vi "Logging List Tree Items.vi"(3 "TreeRef":refnum<vi>) -> (0 "Items":string[](array[string]), 1 "TreeRef":refnum<vi>)   [LabVIEW 2012, in "femtoRoboLib.lvlib"]
uses:
  femtoRoboLib.lvlib
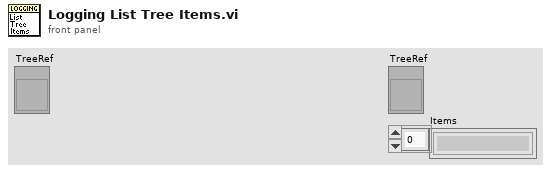
[diagram p1: front panel]
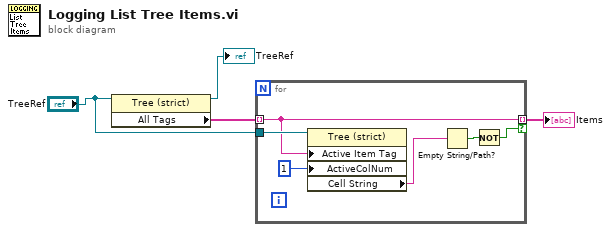
[diagram p0: block diagram]
diagram:
  n1 = property class="Tree (strict)"(reference="TreeRef") -> (reference out=→"TreeRef":refnum<vi>, "All Tags"=w3:string[])  [unwired: 1 in, 1 out]
  n2 = for {
    tunnel: w3 -> [w9] mode=indexing
    tunnel: [w9] -> w2 mode=indexing if=w5
    tunnel: "TreeRef" -> [w10]
    n3 = property class="Tree (strict)"(reference=w10, "Active Item Tag"=w9, "ActiveColNum"=1 ("Active Cell:Active Column Number")) -> ("Cell String"=w7:string)  [unwired: 1 in, 2 out]
    n4 = Empty String/Path?(string/path=w7) -> (empty?=w6:bool)
    n5 = Not(x=w6) -> (.not. x?=w5:bool)
  }
  "Items" <- w2
